vi "Images.vi"() -> ()   [LabVIEW 2019]
uses:
  Classes/Parse/ParseXML/Path.ctl
  Classes/Parse/ParseXML/ParseSVG.lvclass
panel:
  out "Array 2":T1[](array[typedef])
  out "text":string
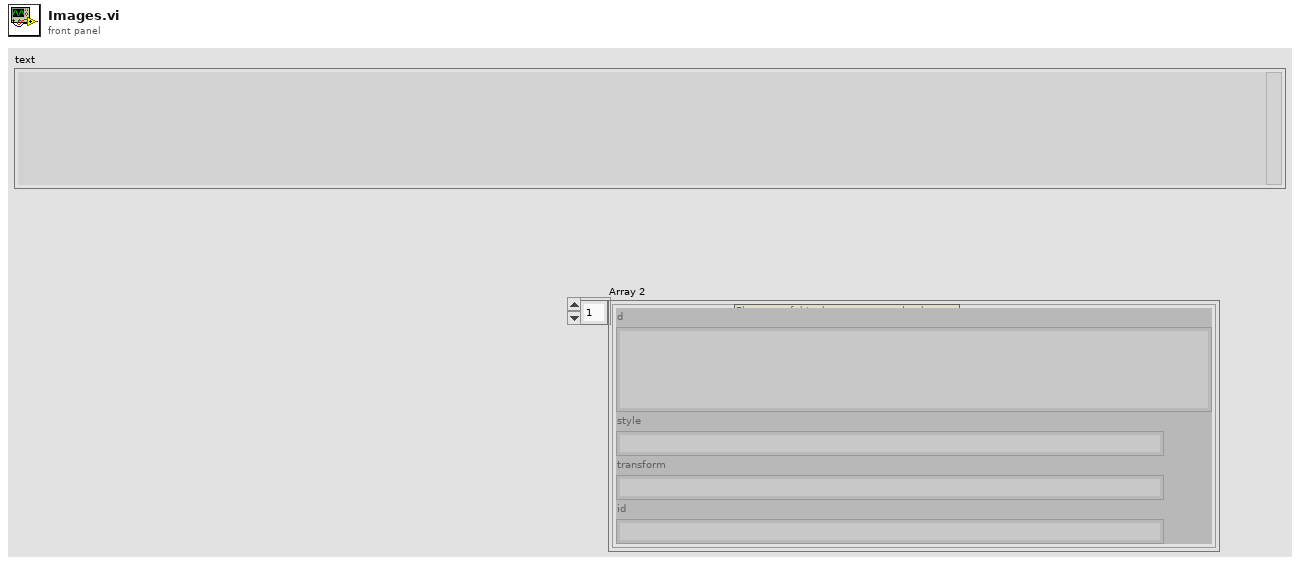
[diagram p1: front panel]
types:
  T1 = typedef "ParseSVG.lvclass/Path.ctl" = cluster{"d":string, "style":string, "transform":string, "id":string}
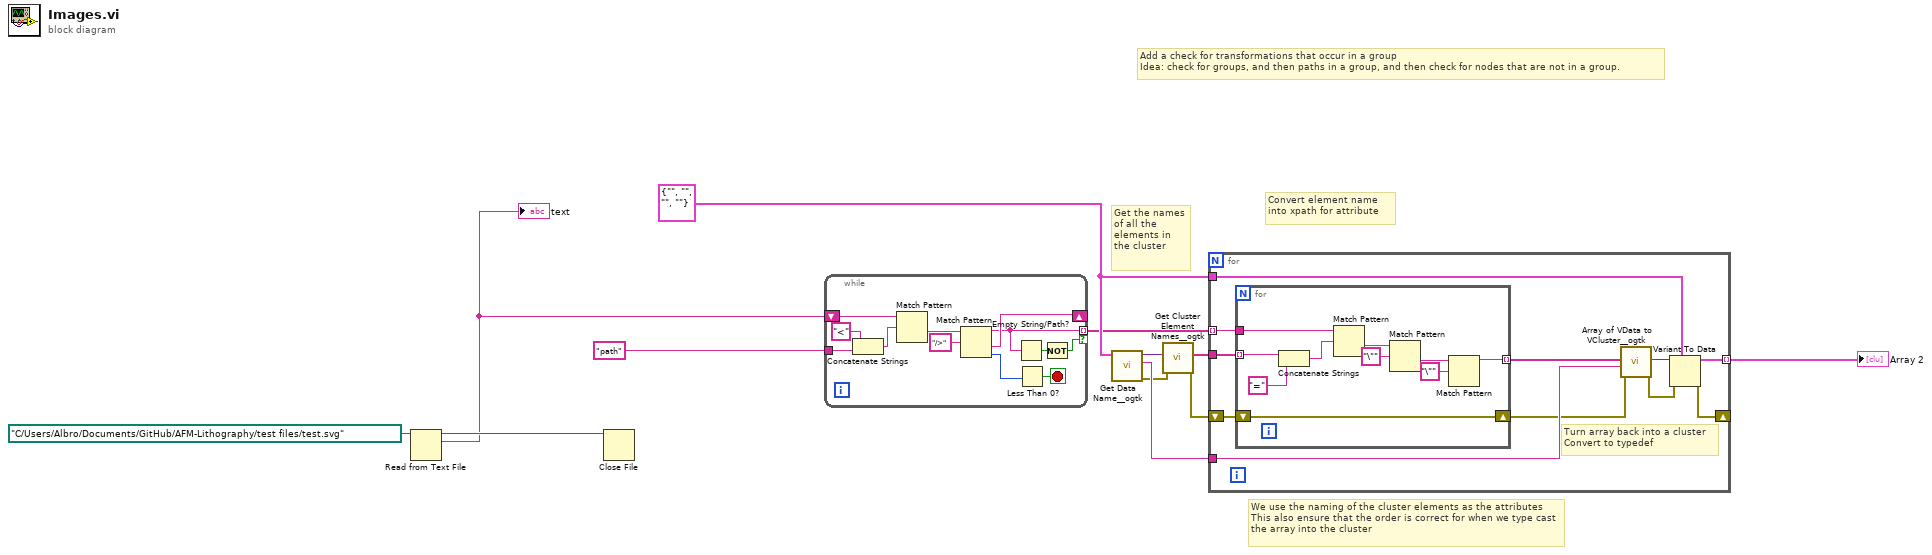
[diagram p0: block diagram]
diagram:
  w4 = T1 {"d"="", "style"="", "transform"="", "id"=""} ("Path")
  # "Add a check for transformations that occur in a group\nIdea: check for groups, and then paths in a group, and then check for nodes that are not in a group."
  # "We use the naming of the cluster elements as the attributes\nThis also ensure that the order is correct for when we type cast the array into the cluster"
  # "Convert element name into xpath for attribute"
  # "Get the names of all the elements in the cluster"
  n1 = Read from Text File(file (use dialog)=path "C:/Users/Albro/Documents/GitHub/AFM-Lithography/test files/test.svg") -> (refnum out=w12:refnum<file>, text=w1:string)  [unwired: 3 in, 2 out]
  "text" <- w1
  n2 = Close File(refnum=w12) -> ()  [unwired: 1 in, 2 out]
  n3 = while {
    shift-right: [w17] -> _
    shift-left: w1 -> [w24]
    tunnel: "path" -> [w23]
    tunnel: [w15] -> w3 mode=indexing if=w16
    stop <- w19 stop-if-true
    n4 = Concatenate Strings("<" ("regular expression"), w23) -> (w22:string)
    n5 = Match Pattern(string=w24, regular expression=w22) -> (after substring=w21:string)  [unwired: 1 in, 3 out]
    n6 = Match Pattern(string=w21, regular expression="/>") -> (before substring=w15:string, after substring=w17:string, offset past match=w14:i32)  [unwired: 1 in, 1 out]
    n7 = Empty String/Path?(string/path=w15) -> (empty?=w18:bool)
    n8 = Less Than 0?(x=w14) -> (x < 0?=w19:bool)
    n9 = Not(x=w18) -> (.not. x?=w16:bool)
  }
  n10 = call <userlib>:"Get Data Name__ogtk.vi"("Data"=w4) -> ("error out"=w5:errorcluster, "Data Name"=w9:string, "Data dup"=w8:variant)  [unwired: 8 in]
  n11 = call <userlib>:"Get Cluster Element Names__ogtk.vi"("error in (no error)"=w5, "Cluster"=w8) -> ("error out"=w6:errorcluster, "Element Names"=w7:string[])  [unwired: 8 in]
  n12 = for {
    shift-right: [w34] -> _
    shift-left: w6 -> [w33]
    tunnel: [w32] -> w2 mode=indexing
    tunnel: w7 -> [w29]
    tunnel: w9 -> [w28]
    tunnel: w4 -> [w27]
    tunnel: w3 -> [w25] mode=indexing
    # "Turn array back into a cluster\nConvert to typedef"
    n13 = for {
      shift-right: [w45] -> w26
      shift-left: w33 -> [w45]
      tunnel: [w39] -> w31 mode=indexing
      tunnel: w29 -> [w37] mode=indexing
      tunnel: w25 -> [w44]
      n14 = Concatenate Strings(w37, "=" ("string")) -> (w38:string)
      n15 = Match Pattern(string=w44, regular expression=w38) -> (after substring=w43:string)  [unwired: 1 in, 3 out]
      n16 = Match Pattern(string=w43, regular expression="\"") -> (after substring=w41:string)  [unwired: 1 in, 3 out]
      n17 = Match Pattern(string=w41, regular expression="\"") -> (before substring=w39:string)  [unwired: 1 in, 3 out]
    }
    n18 = call <userlib>:"Array of VData to VCluster__ogtk.vi"("error in (no error)"=w26, "Cluster Name"=w28, "Array"=w31) -> ("error out"=w35:errorcluster, "VCluster"=w30:variant)  [unwired: 7 in]
    n19 = Variant To Data(error in=w35, type=w27, Variant=w30) -> (data=w32:T1, error out=w34:errorcluster)
  }
  "Array 2" <- w2
